vi "Add Available Measurement.vi"(8 "error in (no error)":errorcluster, 10 "Name":string, 11 "Common Measurements in":refnum<class "Common Measurements.lvclass">) -> (0 "error out":errorcluster, 3 "Common Measurements out":refnum<class "Common Measurements.lvclass">)   [LabVIEW 2015, in "Common Measurements.lvclass"]
uses:
  Common Measurements.lvclass
  Mag Lab Measure Base/Mag Lab Measure Base.lvclass/Mag Lab Measure Base.ctl
  Common Measurements Interface Messages/Add Menu Measurement Msg/Add Menu Measurement Msg.lvclass/Add Menu Measurement Msg.ctl
  <vilib>/ActorFramework/Message Enqueuer/Message Enqueuer.lvclass/Message Enqueuer.ctl
  <vilib>/ActorFramework/Message Enqueuer/Enqueue.vi
  <vilib>/ActorFramework/Message Priority Queue/Priority Enqueue.vi
  Mag Lab Measure Controller/Mag Lab Measure Controller.lvclass
  <vilib>/ActorFramework/Message Enqueuer/Message Enqueuer.lvclass
  Common Measurements Interface Messages/Add Menu Measurement Msg/Add Menu Measurement Msg.lvclass
  Mag Lab Measure Base/Mag Lab Measure Base.lvclass
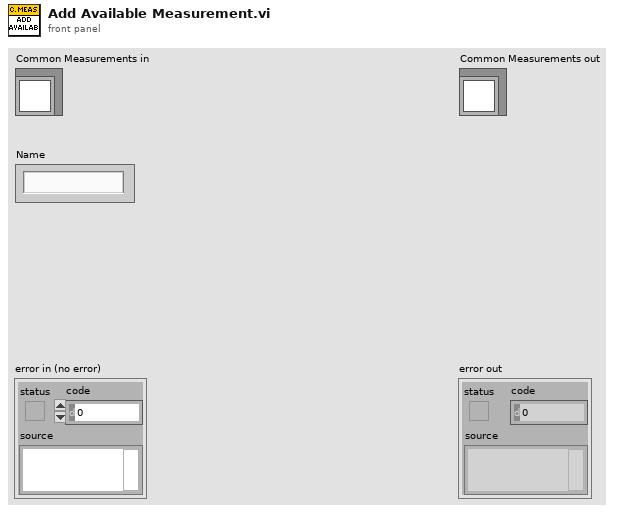
[diagram p1: front panel]
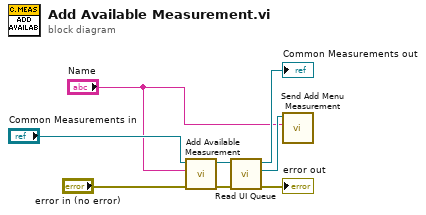
[diagram p0: block diagram]
diagram:
  n1 = call-parent "Add Available Measurement.vi"("error in (no error)"="error in (no error)", "Mag Lab Measurement"="Name", "Mag Lab Measure Controller in"="Common Measurements in") -> ("error out"=w4:errorcluster, "Mag Lab Measure Controller out"=w7:refnum<class "Common Measurements.lvclass">)  [unwired: 7 in]
  n2 = call "Read UI Queue.vi"("error in (no error)"=w4, "Mag Lab Measure Base in"=w7) -> ("error out"=→"error out":errorcluster, "Actor Framework.lvlib:Message Enqueuer"=w5:refnum<class "Message Enqueuer.lvclass">, "Mag Lab Measure Base out"=→"Common Measurements out":refnum<class "Common Measurements.lvclass">)  [unwired: 7 in]
  n3 = call "Send Add Menu Measurement.vi"("Name"="Name", "Message Enqueuer"=w5) -> ()  [unwired: 8 in, 2 out]
